vi "Data Log Fetcher.vi"() -> ()   [LabVIEW 2013]
uses:
  <vilib>/measure/maresamp.llb/Resample N Waveforms (single shot).vi
  <vilib>/Waveform/WDTFileIO.llb/ Write Waveforms to File (1D).vi
  <vilib>/Waveform/WDTFileIO.llb/Export Waveforms To Spreadsheet File (1D).vi
  <vilib>/httpClient/LabVIEWHTTPClient.lvlib
  Data Log Fetcher.lvlib
  <vilib>/measure/NI_MAPro.lvlib
panel:
  in  "Image Path 2":path
  in  "Write to PNG 2":bool
  out "Waveform Graph 2":waveform(dbl)[](graph)
  in  "Image Path":path
  in  "Write to PNG":bool
  in  "Resample dt":u32
  out "Device":string
  in  "Write to CSV":bool
  in  "Write to WFM":bool
  out "Data Logger Output":string
  in  "Device Display Index":u32=1
  out "Waveform Graph":waveform(dbl)(graph)
  out "Parsing":bool
  out "Fetching":bool
  out "Raw Data":dbl[][][](array[numeric])
  out "Fetch Command URL":string
  in  "Fetch":bool
  in  "stop":bool
  in  "End Time":timestamp=timestamp(3509586000 s since 1904-01-01)
  in  "Start Time":timestamp=timestamp(3509586000 s since 1904-01-01)
  in  "Number to Skip":u32
  in  "Devices List":string="e:201vac,e:c2ctpr,e:c2cbig,e:c2frg1,e:solig2,e:c2cbpr,e:c2clig,e:c2crig,e:c2clpr,e:c2crpr,e:c2frg2,e:c2wmig,e:c2prob"
  # "e:mtamr1,e:mtamr2,e:mtamr3,e:mtamr4"
  # "number of points to skip before returning one"
  # "Separate device names by a comma."
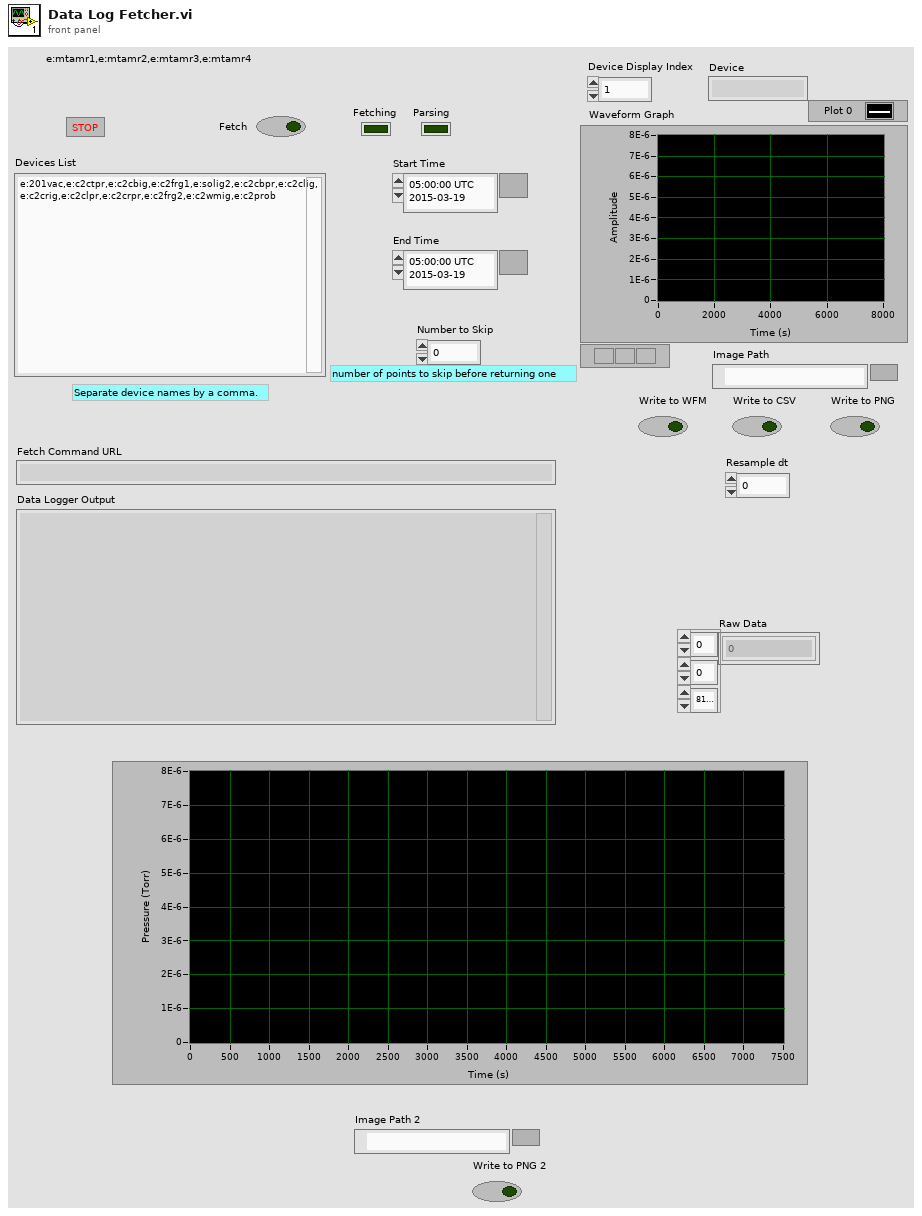
[diagram p1: front panel]
types:
  T1 = typedef "imagedata.ctl" = cluster{"image type":i32, "image depth":i32, "image":u8[], "mask":u8[], "colors":u32[], "Rectangle":cluster{"left":i16, "top":i16, "right":i16, "bottom":i16}}
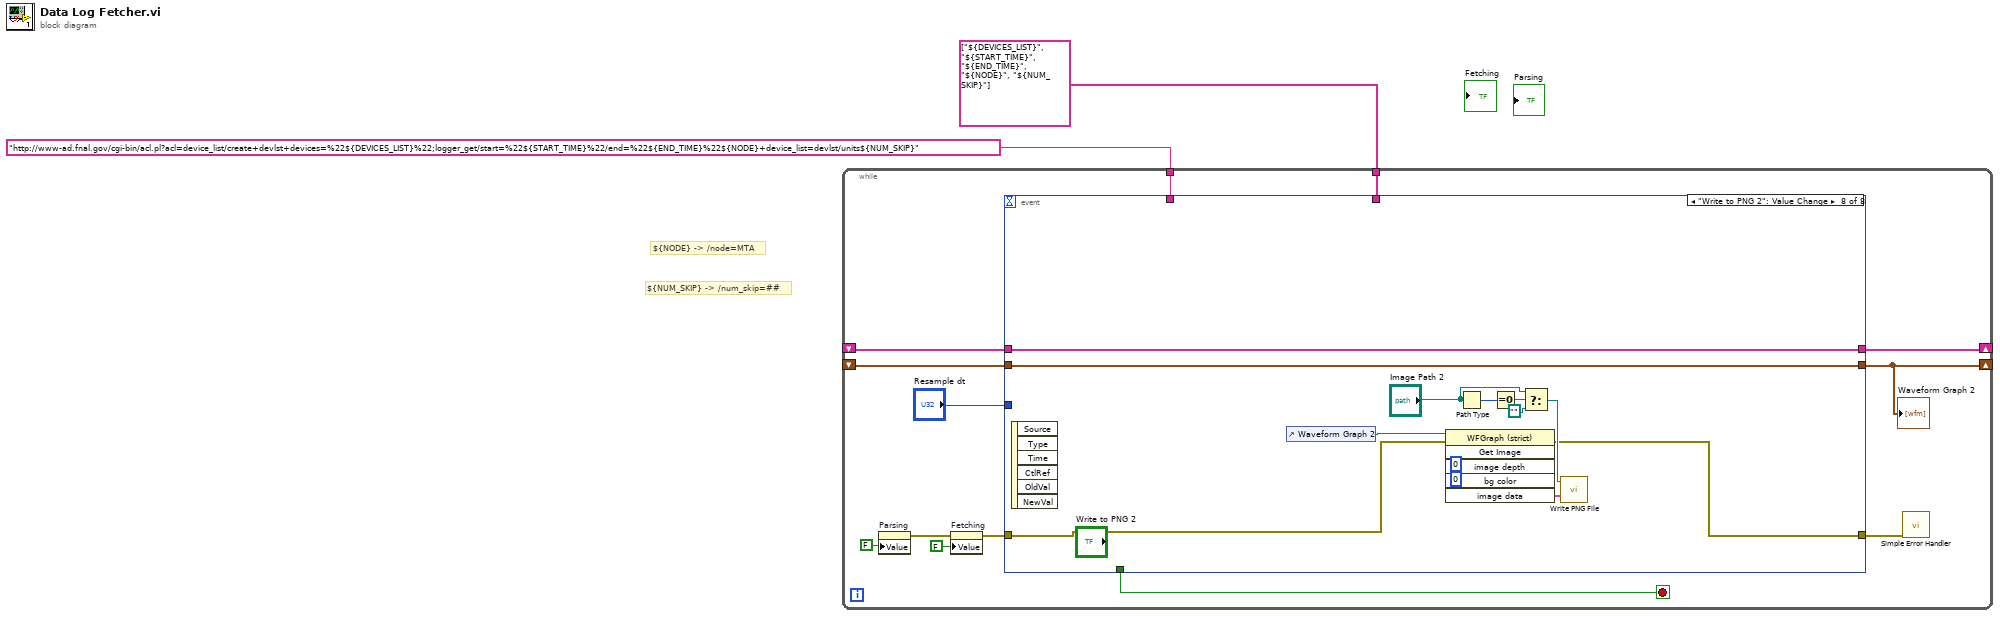
[diagram p0: block diagram]
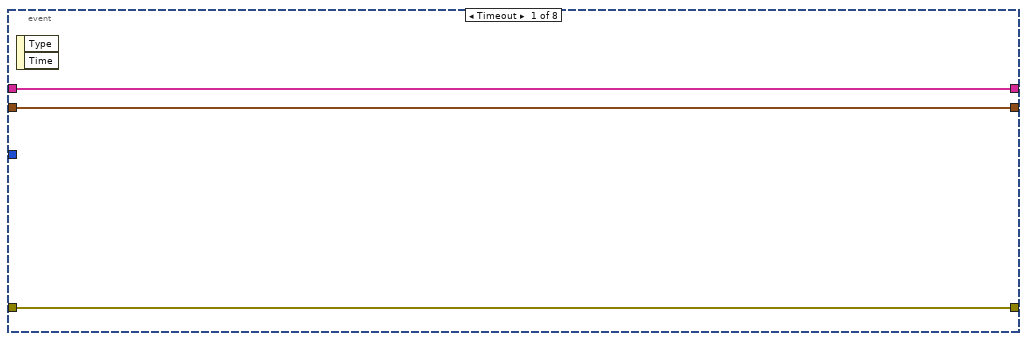
[diagram p2: hidden frame]
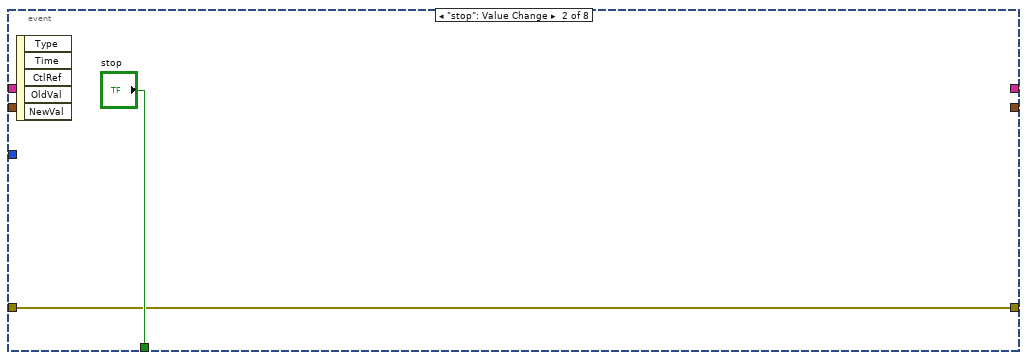
[diagram p3: hidden frame]
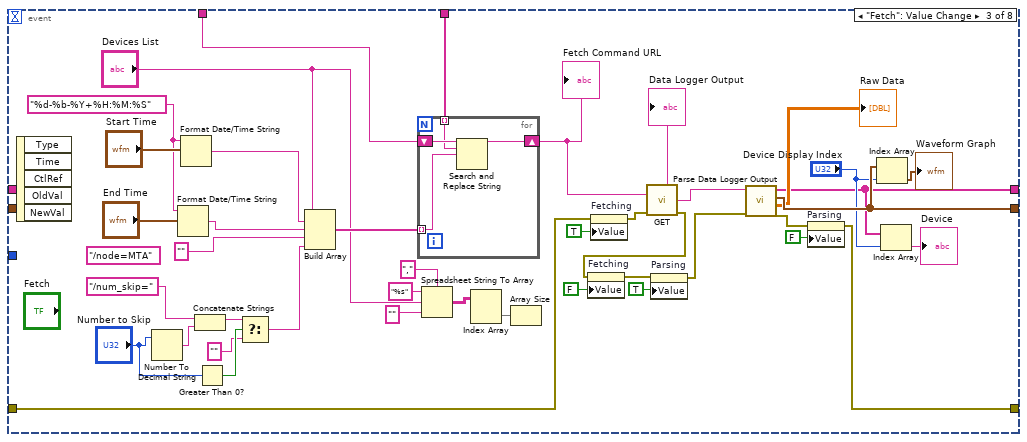
[diagram p4: hidden frame]
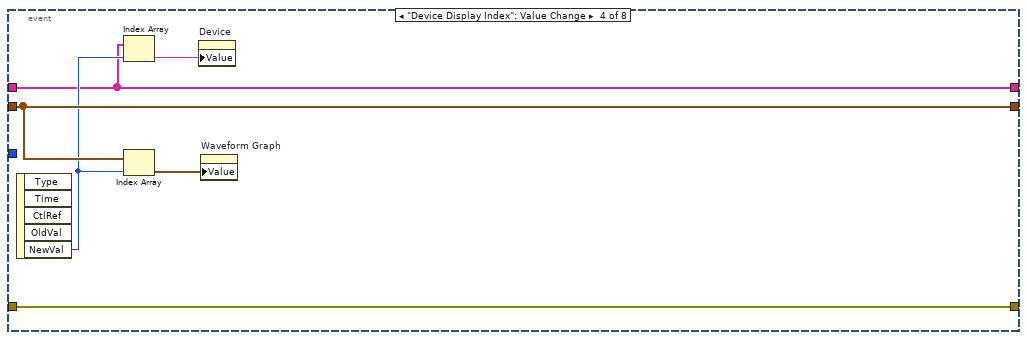
[diagram p5: hidden frame]
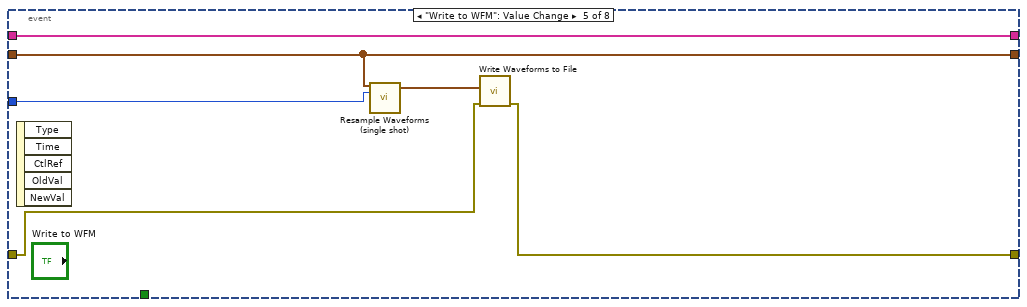
[diagram p6: hidden frame]
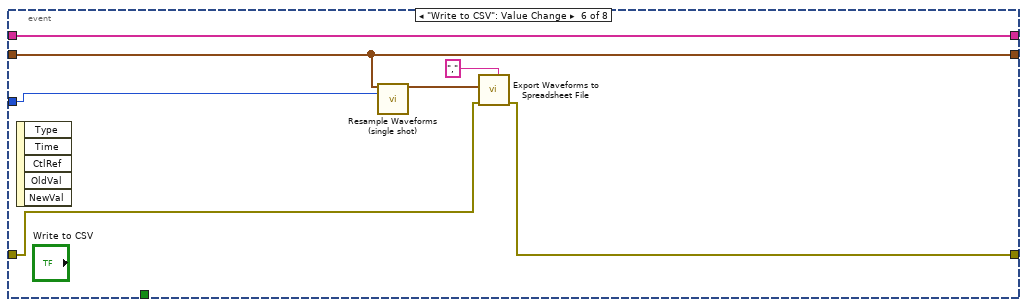
[diagram p7: hidden frame]
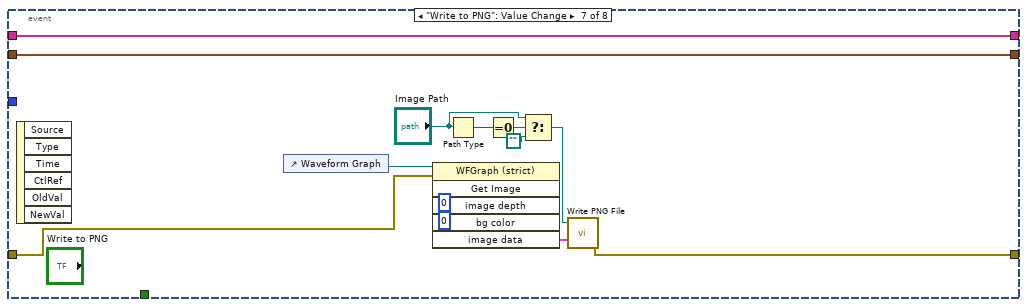
[diagram p8: hidden frame]
diagram:
  # "${NUM_SKIP} -> /num_skip=##"
  # "${NODE} -> /node=MTA"
  n1 = while {
    tunnel: "http://www-ad.fnal.gov/cgi-bin/acl.pl?acl=device_list/create+devlst+devices=%22${DEVICES_LIST}%22;logger_get/start=%22${START_TIME}%22/end=%22${END_TIME}%22${NODE}+device_list=devlst/units${NUM_SKIP}" -> [w14]
    tunnel: string[] ["${DEVICES_LIST}", "${START_TIME}", "${END_TIME}", "${NODE}", "${NUM_SKIP}"] -> [w13]
    shift-right: [w3] -> _
    shift-left: _ -> [w8]
    shift-right: [w6] -> _
    shift-left: _ -> [w5]
    stop <- w15 stop-if-true
    n2 = property on="Parsing" class="Bool (strict)"("Value"=FALSE ("Parsing")) -> (error out=w12:errorcluster)  [unwired: 2 in, 1 out]
    n3 = property on="Fetching" class="Bool (strict)"(error in=w12, "Value"=FALSE ("Fetching")) -> (error out=w9:errorcluster)  [unwired: 1 in, 1 out]
    n4 = event shown="[7] \"Write to PNG 2\": Value Change" {
      selector: _ -> [_ _ _ _ _ _ _ _]
      dyn-events: _ -> [_ _ _ _ _ _ _ _]
      timeout: _ -> [_ _ _ _ _ _ _ _]
      tunnel: [_ "stop" _ _ _ _ _ _] -> w15
      tunnel: w14 -> [_ _ w47 _ _ _ _ _]
      tunnel: w13 -> [_ _ w48 _ _ _ _ _]
      tunnel: w9 -> [w17 w19 w29 w69 w77 w84 w88 w101]
      tunnel: [w18 _ w26 w70 w74 w80 w85 w98] -> w3
      tunnel: w8 -> [w18 _ _ w70 w74 w80 w85 w98]
      tunnel: [w17 w19 w24 w69 w76 w83 w87 w100] -> w7
      tunnel: [w16 _ w21 w66 w75 w81 w86 w99] -> w6
      tunnel: w5 -> [w16 _ _ w66 w75 w81 w86 w99]
      tunnel: "Resample dt" -> [_ _ _ _ w72 w78 _ _]
      event Timeout {
        n5 = event-data() -> ()  [unwired: 1 in, 2 out]
      }
      event "stop": Value Change {
        n6 = event-data() -> ()  [unwired: 1 in, 5 out]
      }
      event "Fetch": Value Change {
        w59 = "%d-%b-%Y+%H:%M:%S" ("time format string (%c)")
        (unwired) "/node=MTA"
        n7 = event-data() -> ()  [unwired: 1 in, 5 out]
        n8 = Number To Decimal String(number="Number to Skip") -> (decimal integer string=w57:string)  [unwired: 1 in]
        n9 = Format Date/Time String(time format string (%c)=w59, seconds (now)="End Time") -> (date/time string=w51:string)  [unwired: 1 in]
        n10 = Format Date/Time String(time format string (%c)=w59, seconds (now)="Start Time") -> (date/time string=w50:string)  [unwired: 1 in]
        n11 = Concatenate Strings("/num_skip=", w57) -> (w54:string)
        n12 = Greater Than 0?(x="Number to Skip") -> (x > 0?=w55:bool)
        n13 = Select(t=w54, s=w55, f="") -> (s? t:f=w52:string)
        n14 = Build Array("Devices List", w50, w51, "" ("element"), w52) -> (w49:string[])
        n15 = for {
          tunnel: w49 -> [w62] mode=indexing
          tunnel: w48 -> [w63] mode=indexing
          shift-right: [w64] -> w46
          shift-left: w47 -> [w65]
          n16 = Search and Replace String(input string=w65, search string=w63, replace string=w62) -> (result string=w64:string)  [unwired: 5 in, 3 out]
        }
        "Fetch Command URL" <- w46
        n17 = Spreadsheet String To Array(delimiter (Tab)=",", format string="%s", spreadsheet string="Devices List", array type (2D Dbl)="" ("delimiter (Tab)")) -> (array=w40:string[][])
        n18 = Index Array(array=w40) -> (element=w39:string[])  [unwired: 2 in]
        n19 = Array Size(array=w39) -> ()  [unwired: 1 out]
        n20 = property on="Fetching" class="Bool (strict)"(error in=w29, "Value"=TRUE ("Fetching")) -> (error out=w38:errorcluster)  [unwired: 1 in, 1 out]
        n21 = call <vilib>:"GET.vi"("url"=w46, "error in (no error)"=w38) -> ("body"=w45:string, "error out"=w35:errorcluster)  [unwired: 10 in, 2 out]
        "Data Logger Output" <- w45
        n22 = property on="Fetching" class="Bool (strict)"(error in=w35, "Value"=FALSE ("Fetching")) -> (error out=w34:errorcluster)  [unwired: 1 in, 1 out]
        n23 = property on="Parsing" class="Bool (strict)"(error in=w34, "Value"=TRUE ("Parsing")) -> (error out=w32:errorcluster)  [unwired: 1 in, 1 out]
        n24 = call "Parse Data Logger Output.vi"("error in"=w32, "Data Logger Output"=w45) -> ("error out"=w30:errorcluster, "Raw Data"=→"Raw Data":dbl[][][], "Resampled Data"=w26:waveform(dbl)[], "Device List"=w21:string[])  [unwired: 6 in]
        n25 = property on="Parsing" class="Bool (strict)"(error in=w30, "Value"=FALSE ("Parsing")) -> (error out=w24:errorcluster)  [unwired: 1 in, 1 out]
        n26 = Index Array(array=w26, index="Device Display Index") -> (element=→"Waveform Graph":waveform(dbl))
        n27 = Index Array(array=w21, index="Device Display Index") -> (element=→"Device":string)
      }
      event "Device Display Index": Value Change {
        n28 = event-data() -> ("NewVal"=w67:u32)  [unwired: 1 in, 4 out]
        n29 = Index Array(array=w66, index=w67) -> (element=w68:string)
        n30 = Index Array(array=w70, index=w67) -> (element=w71:waveform(dbl))
        n31 = property on="Device" class="Str"("Value"=w68) -> ()  [unwired: 2 in, 2 out]
        n32 = property on="Waveform Graph" class="WFGraph (strict)"("Value"=w71) -> ()  [unwired: 2 in, 2 out]
      }
      event "Write to WFM": Value Change {
        n33 = event-data() -> ()  [unwired: 1 in, 5 out]
        n34 = call-poly <vilib>:"Resample Waveforms (single shot).vi"("waveforms in"=w74, "dt"=w72) -> ("resampled waveforms out"=w73:waveform(dbl)[])  [unwired: 10 in, 3 out]
        n35 = call-poly <vilib>:"Write Waveforms to File.vi"("error in (no error)"=w77, "waveform array"=w73) -> ("error out"=w76:errorcluster)  [unwired: 8 in, 1 out]
      }
      event "Write to CSV": Value Change {
        n36 = event-data() -> ()  [unwired: 1 in, 5 out]
        n37 = call-poly <vilib>:"Resample Waveforms (single shot).vi"("waveforms in"=w80, "dt"=w78) -> ("resampled waveforms out"=w79:waveform(dbl)[])  [unwired: 10 in, 3 out]
        n38 = call-poly <vilib>:"Export Waveforms to Spreadsheet File.vi"("delimiter (Tab)"=",", "error in (no error)"=w84, "waveforms"=w79) -> ("error out"=w83:errorcluster)  [unwired: 7 in, 1 out]
      }
      event "Write to PNG": Value Change {
        n39 = event-data() -> ()  [unwired: 1 in, 6 out]
        n40 = control-ref of="Waveform Graph"() -> (w89:refnum<vi>)
        n41 = invoke on="Invoke Node" class="WFGraph (strict)" method="Get Image"(reference=w89, error in=w88, "image depth"=0 ("Image Depth"), "bg color"=u32 0 ("Background Color")) -> ("image data"=w95:T1)  [unwired: 2 in, 5 out]
        n42 = Path Type(1:"Image Path") -> (0:w94:i16)
        n43 = Equal To 0?(x=w94) -> (x = 0?=w93:bool)
        n44 = Select(t="Image Path", s=w93, f=path "") -> (s? t:f=w92:path)
        n45 = call <vilib>:"Write PNG File.vi"("image data"=w95, "path to PNG file"=w92) -> ("error out"=w87:errorcluster)  [unwired: 8 in, 1 out]
      }
      event "Write to PNG 2": Value Change {
        n46 = event-data() -> ()  [unwired: 1 in, 6 out]
        n47 = control-ref of="Waveform Graph 2"() -> (w102:refnum<vi>)
        n48 = invoke on="Invoke Node" class="WFGraph (strict)" method="Get Image"(reference=w102, error in=w101, "image depth"=0 ("Image Depth"), "bg color"=u32 0 ("Background Color")) -> (error out=w100:errorcluster, "image data"=w107:T1)  [unwired: 2 in, 4 out]
        n49 = Path Type(1:"Image Path 2") -> (0:w106:i16)
        n50 = Equal To 0?(x=w106) -> (x = 0?=w105:bool)
        n51 = Select(t="Image Path 2", s=w105, f=path "") -> (s? t:f=w104:path)
        n52 = call <vilib>:"Write PNG File.vi"("image data"=w107, "path to PNG file"=w104) -> ()  [unwired: 8 in, 2 out]
      }
    }
    "Waveform Graph 2" <- w3
    n53 = call <vilib>:"Simple Error Handler.vi"("error in (no error)"=w7) -> ()  [unwired: 4 in, 5 out]
  }
